vi "format.vi"() -> ()   [LabVIEW 2020]
panel:
  out "output 3":dbl
  out "output 2":dbl
  out "output 1":dbl
  out "resulting string":string
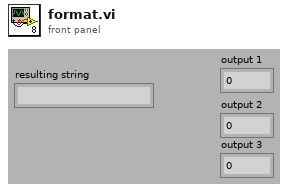
[diagram p1: front panel]
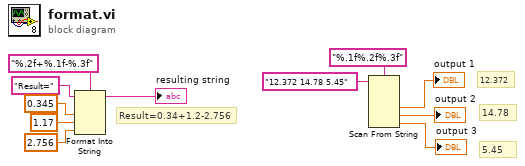
[diagram p0: block diagram]
diagram:
  # "5.45"
  # "14.78"
  # "12.372"
  # "Result=0.34+1.2-2.756"
  n1 = Format Into String "Format Into String"(format string="%.2f+%.1f-%.3f", initial string="Result=", 0.345 ("input 1"), 1.17 ("input 2"), 2.756 ("input 3")) -> (resulting string=→"resulting string":string)  [unwired: 1 in, 1 out]
  n2 = Scan From String(format string="%.1f%.2f%.3f", input string="12.372 14.78 5.45") -> (output 1=→"output 1":dbl, output 2=→"output 2":dbl, output 3=→"output 3":dbl)  [unwired: 2 in, 6 out]
